vi "Create Plugin Directories.vi"(8 "error in (no error)":errorcluster, 11 "Plugin Directory Array":path[](array[path])) -> (0 "error out":errorcluster, 3 "Creation Success":bool[](array[boolean]))   [LabVIEW 2020, in "Plugin Manager.lvlib"]
uses:
  Plugin Manager.lvlib
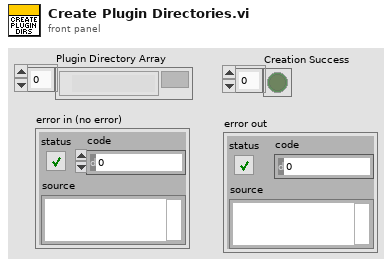
[diagram p1: front panel]
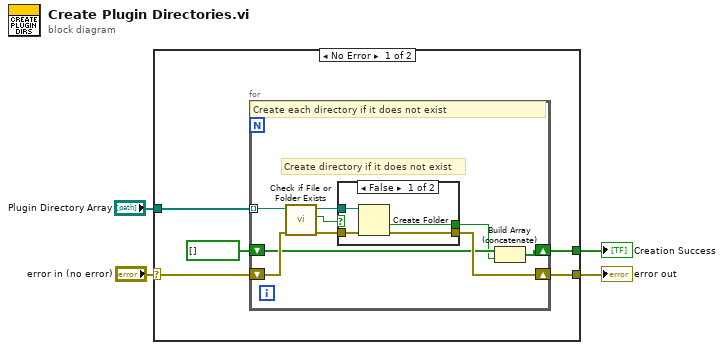
[diagram p0: block diagram]
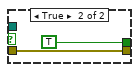
[diagram p2: hidden frame]
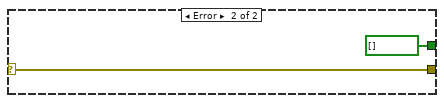
[diagram p3: hidden frame]
diagram:
  n1 = case shown="No Error" "error in (no error)" {
    selector: "error in (no error)" -> [w6 w25]
    tunnel: "Plugin Directory Array" -> [w9 _]
    tunnel: [w8 w25] -> w3
    tunnel: [w5 bool[] []] -> w1
    frame No Error {
      n2 = for {
        tunnel: w9 -> [w17] mode=indexing
        shift-right: [w18] -> w8
        shift-left: w6 -> [w15]
        shift-right: [w12] -> w5
        shift-left: bool[] [] -> [w13]
        # "Create directory if it does not exist"
        # "Create each directory if it does not exist"
        n3 = call <vilib>:"Check if File or Folder Exists.vi"("error in (no error)"=w15, "path"=w17) -> ("error out"=w14:errorcluster, "file or folder exists?"=w10:bool, "dup path"=w16:path)  [unwired: 7 in]
        n4 = case shown="False" w10 {
          tunnel: [w22 w24] -> w18
          tunnel: w16 -> [w21 _]
          tunnel: w14 -> [w20 w24]
          tunnel: [w19 TRUE ("cancelled")] -> w11
          frame False {
            n5 = Create Folder(path (use dialog)=w21, error in=w20) -> (cancelled=w19:bool, error out=w22:errorcluster)  [unwired: 1 in, 1 out]
          }
          frame True {
          }
        }
        n6 = Build Array (concatenate)(w13, w11) -> (w12:bool[])
      }
    }
    frame Error {
    }
  }
  "error out" <- w3
  "Creation Success" <- w1
